vi "PH_Beckhoff_PP_PU.handle PSUs.vi"(0 "i ref in":refnum<vi>, 4 "Values":T2, 5 "error in":errorcluster, 7 "Values changed at":T1) -> (14 "i ref out":refnum<vi>, 19 "error out":errorcluster)   [LabVIEW 2014, in "PH_Beckhoff_PP_PU.lvlib"]
doc: "This VI handles the incoming information about PSU inputs: The status is calculated and, if it changed, set to own attributes and published via DIM. All information is indicated at the GUI."
uses:
  PH_Beckhoff_PP_PU.lvlib
  PH_Beckhoff/PH_Beckhoff.Values.ctl
  PH_Beckhoff/PH_Beckhoff.Sonderklemmen Inputs.ctl
  PH_Beckhoff/PH_Beckhoff.Analog Inputs.ctl
  PH_Beckhoff/PH_Beckhoff.Scaling Type.ctl
  PH_Beckhoff/PH_Beckhoff.Analog Outputs.ctl
  PH_Beckhoff/PH_Beckhoff.Digital Inputs.ctl
  PH_Beckhoff/PH_Beckhoff.Digital Outputs.ctl
  PH_Beckhoff/PH_Beckhoff.lvlib
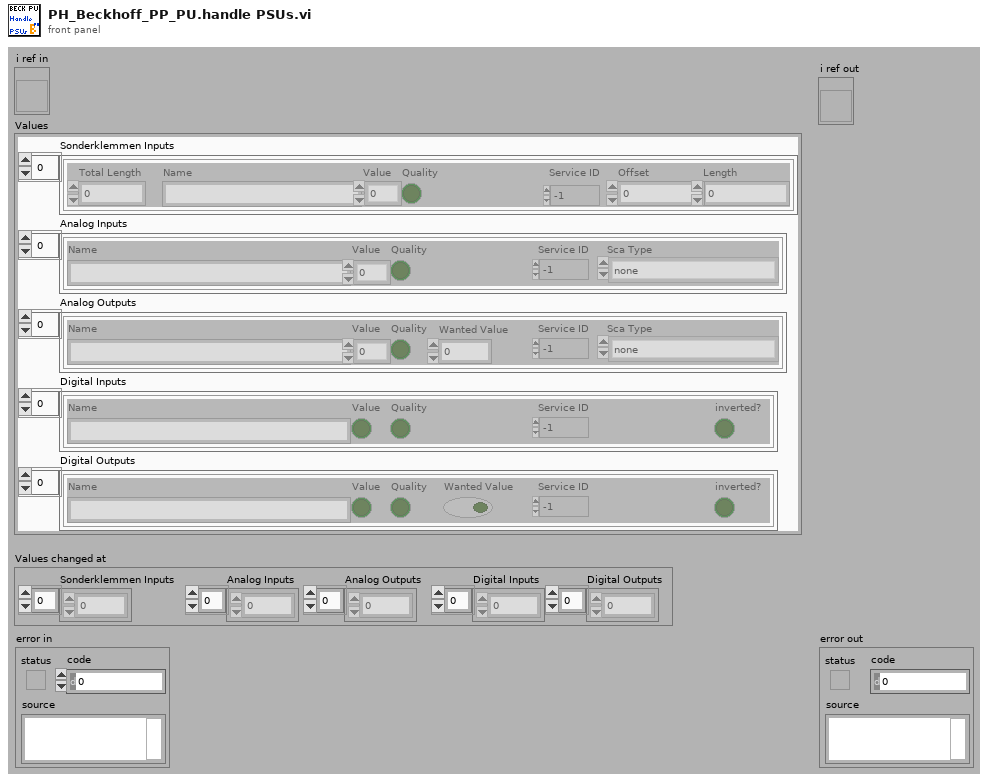
[diagram p1: front panel]
types:
  T1 = cluster{"Sonderklemmen Inputs":i32[], "Analog Inputs":i32[], "Analog Outputs":i32[], "Digital Inputs":i32[], "Digital Outputs":i32[]}
  T2 = typedef "PH_Beckhoff.lvlib/PH_Beckhoff.Values.ctl" = cluster{"Sonderklemmen Inputs":T3, "Analog Inputs":T4, "Analog Outputs":T6, "Digital Inputs":T7, "Digital Outputs":T8}
  T3 = typedef "PH_Beckhoff.lvlib/PH_Beckhoff.Sonderklemmen Inputs.ctl" = cluster{"Total Length":u32, "Name":string, "Value":u64, "Quality":bool, "Service ID":i32, "Offset":u32, "Length":u32}[]
  T4 = typedef "PH_Beckhoff.lvlib/PH_Beckhoff.Analog Inputs.ctl" = cluster{"Name":string, "Value":u32, "Quality":bool, "Service ID":i32, "Sca Type":T5}[]
  T5 = typedef "PH_Beckhoff.lvlib/PH_Beckhoff.Scaling Type.ctl" = enum16{"none", "0 ... 15 Bit -> 0 ... 5", "0 ... 15 Bit -> 0 ... 10", "0 ... 15 Bit -> 0 ... 25", "0 ... 15 Bit -> 4 ... 20", "0 ... 15 Bit -> 0 ... 1", "0 ... 15 Bit -> 0 ... 20000", "0 ... 15 Bit -> 0 ... 24000"}
  T6 = typedef "PH_Beckhoff.lvlib/PH_Beckhoff.Analog Outputs.ctl" = cluster{"Name":string, "Value":u32, "Quality":bool, "Wanted Value":u32, "Service ID":i32, "Sca Type":T5}[]
  T7 = typedef "PH_Beckhoff.lvlib/PH_Beckhoff.Digital Inputs.ctl" = cluster{"Name":string, "Value":bool, "Quality":bool, "Service ID":i32, "inverted?":bool}[]
  T8 = typedef "PH_Beckhoff.lvlib/PH_Beckhoff.Digital Outputs.ctl" = cluster{"Name":string, "Value":bool, "Quality":bool, "Wanted Value":bool, "Service ID":i32, "inverted?":bool}[]
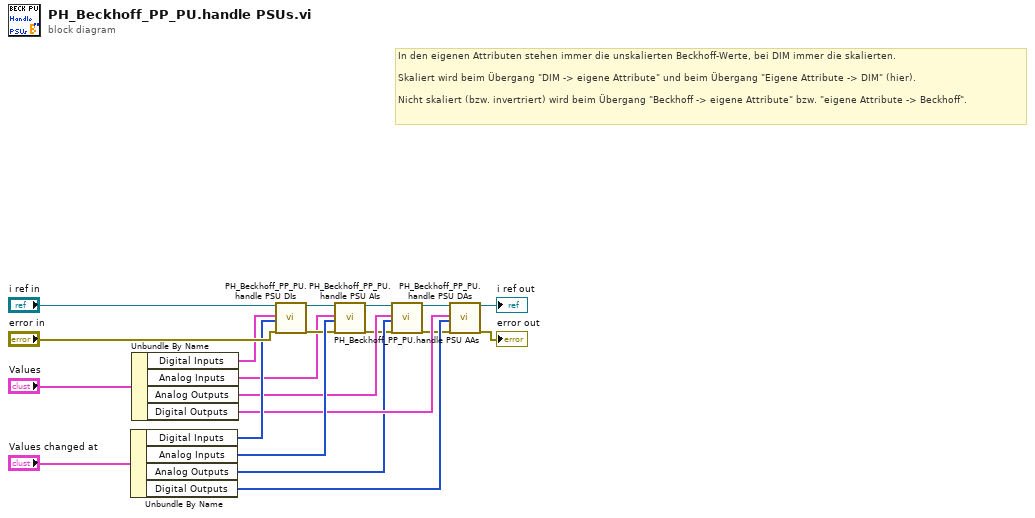
[diagram p0: block diagram]
diagram:
  # "In den eigenen Attributen stehen immer die unskalierten Beckhoff-Werte, bei DIM immer die skalierten.\n\nSkaliert wird beim Übergang \"DIM -> eigene Attribute\" und beim Übergang \"Eigene Attribute -> DIM\" (hier).\n\nNicht skaliert (bzw. invertriert) wird beim Übergang \"Beckhoff -> eigene Attribute\" bzw. \"eigene Attribute -> Beckhoff\"."
  n1 = Unbundle By Name("Values changed at") -> ("Digital Inputs"=w15:i32[], "Analog Inputs"=w19:i32[], "Analog Outputs"=w7:i32[], "Digital Outputs"=w8:i32[])
  n2 = Unbundle By Name("Values") -> ("Digital Inputs"=w14:T7, "Analog Inputs"=w12:T4, "Analog Outputs"=w9:T6, "Digital Outputs"=w11:T8)
  n3 = call "PH_Beckhoff_PP_PU.handle PSU DIs.vi"("i ref in"="i ref in", "Digital Input Values"=w14, "Changed Digital Inputs"=w15, "error in"="error in") -> ("i ref out"=w13:refnum<vi>, "error out"=w17:errorcluster)  [unwired: 14 in]
  n4 = call "PH_Beckhoff_PP_PU.handle PSU AIs.vi"("i ref in"=w13, "Analog Inputs"=w12, "Changed analog Inputs"=w19, "error in"=w17) -> ("i ref out"=w6:refnum<vi>, "error out"=w5:errorcluster)  [unwired: 14 in]
  n5 = call "PH_Beckhoff_PP_PU.handle PSU AAs.vi"("i ref in"=w6, "Analog Output Values"=w9, "Changed analog Outputs"=w7, "error in"=w5) -> ("i ref out"=w3:refnum<vi>, "error out"=w2:errorcluster)  [unwired: 14 in]
  n6 = call "PH_Beckhoff_PP_PU.handle PSU DAs.vi"("i ref in"=w3, "Digital Output Values"=w11, "Changed digital Outputs"=w8, "error in"=w2) -> ("i ref out"=→"i ref out":refnum<vi>, "error out"=→"error out":errorcluster)  [unwired: 14 in]
